vi "Settings.vi"(4 "StopOnOverflow":bool, 5 "DeviceIndex":i32, 6 "Range No.":i32 min=0 max=5 step=1, 7 "SyncDiv":i32=1 min=1 max=8 step=1, 8 "CFD1 zero X":i32=10 min=0 max=40 step=1, 9 "CFD1 level":i32=50 min=0 max=400 step=1, 10 "CFD0 zero X":i32=10 min=-1300 max=400 step=10, 11 "CFD0 level":i32=50 min=-1300 max=400 step=10) -> (0 "Resolution":i32, 2 "Error":bool)   [LabVIEW 2018]
uses:
  phlib.dll
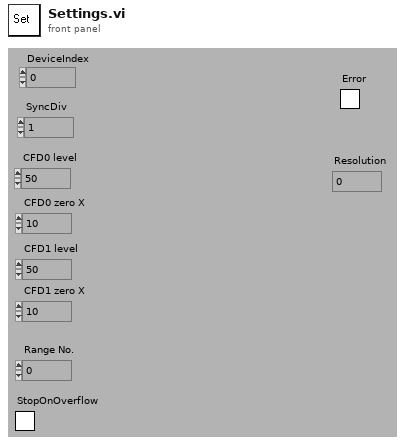
[diagram p1: front panel]
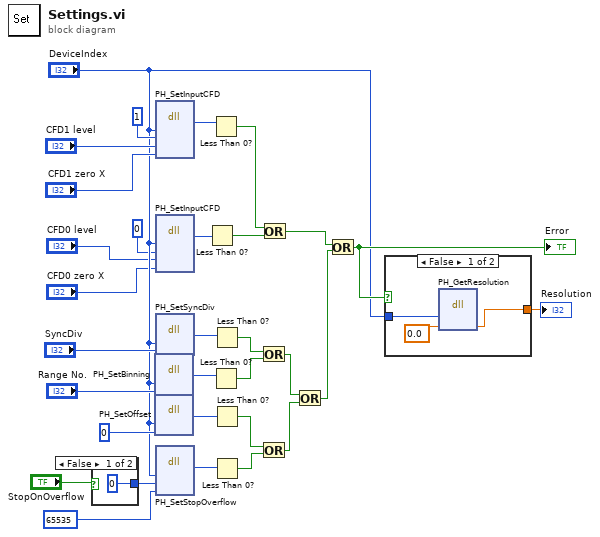
[diagram p0: block diagram]
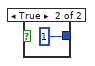
[diagram p2: hidden frame]
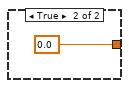
[diagram p3: hidden frame]
diagram:
  n1 = case shown="False" "StopOnOverflow" {
    tunnel: [0 1] -> w10
    frame False {
    }
    frame True {
    }
  }
  n2 = dll-call lib="phlib.dll" fn="PH_SetBinning"("devidx"="DeviceIndex", "Binning"="Range No.") -> (w30:i32)  [unwired: 5 in, 2 out]
  n3 = dll-call lib="phlib.dll" fn="PH_SetOffset"("devidx"="DeviceIndex", "Offset"=0) -> (w28:i32)  [unwired: 5 in, 2 out]
  n4 = dll-call lib="phlib.dll" fn="PH_SetInputCFD"("devidx"="DeviceIndex", "channel"=1, "Level"="CFD1 level", "zerocross"="CFD1 zero X") -> (w31:i32)  [unwired: 7 in, 2 out]
  n5 = dll-call lib="phlib.dll" fn="PH_SetInputCFD"("devidx"="DeviceIndex", "channel"=0, "Level"="CFD0 level", "zerocross"="CFD0 zero X") -> (w3:i32)  [unwired: 7 in, 2 out]
  n6 = dll-call lib="phlib.dll" fn="PH_SetSyncDiv"("devidx"="DeviceIndex", "divider"="SyncDiv") -> (w21:i32)  [unwired: 5 in, 2 out]
  n7 = dll-call lib="phlib.dll" fn="PH_SetStopOverflow"("devidx"="DeviceIndex", "StopOnOfl"=w10, "level"=65535) -> (w25:i32)  [unwired: 6 in, 2 out]
  n8 = Less Than 0?(x=w3) -> (x < 0?=w2:bool)
  n9 = Less Than 0?(x=w31) -> (x < 0?=w29:bool)
  n10 = Less Than 0?(x=w30) -> (x < 0?=w19:bool)
  n11 = Less Than 0?(x=w21) -> (x < 0?=w20:bool)
  n12 = Less Than 0?(x=w28) -> (x < 0?=w24:bool)
  n13 = Less Than 0?(x=w25) -> (x < 0?=w23:bool)
  n14 = Or(x=w20, y=w19) -> (x .or. y?=w18:bool)
  n15 = Or(x=w24, y=w23) -> (x .or. y?=w17:bool)
  n16 = Or(x=w29, y=w2) -> (x .or. y?=w1:bool)
  n17 = Or(x=w18, y=w17) -> (x .or. y?=w16:bool)
  n18 = Or(x=w1, y=w16) -> (x .or. y?=w26:bool)
  "Error" <- w26
  n19 = case shown="False" w26 {
    tunnel: [w34 0.0] -> w27
    tunnel: "DeviceIndex" -> [w36 _]
    frame False {
      n20 = dll-call lib="phlib.dll" fn="PH_GetResolution"("devidx"=w36, "resolution"=0.0) -> ("resolution"=w34:dbl)  [unwired: 5 in, 2 out]
    }
    frame True {
    }
  }
  "Resolution" <- w27
